vi "NIMS_dfd_Convert Band Specs (Remez Ripple).vi"(9 "Ripple":dbl[](array[numeric]), 10 "A":dbl[](array[numeric]), 11 "F":dbl[](array[numeric])) -> (0 "error out":errorcluster, 2 "band specs":T1[](array[typedef])=[{"band specification"=[{"freq"=0.0, "amplitude"=1.0, "weight"=1.0}, {"freq"=0.2, "amplitude"=1.0, "weight"=1.0}], "ripple constraint"=0.0}, {"band specification"=[{"freq"=0.3, "amplitude"=0.0, "weight"=1.0}, {"freq"=0.5, "amplitude"=0.0, "weight"=1.0}], "ripple constraint"=0.0}])   [LabVIEW 2017, in "NI_DigFilter_MathScript.lvlib"]
uses:
  <vilib>/addons/Digital Filter Design/NI_DigFilter_MathScript.lvlib
  <vilib>/addons/Digital Filter Design/_Objects.llb/DFD Adv Band Spec.ctl
  <vilib>/addons/Digital Filter Design/_Misc.llb/dfd_Error Handlers (Multiple).vi
  <vilib>/addons/Digital Filter Design/NI_DigFilterLicensed.lvlib
panel:
  # "freq"
  # "amplitude"
  # "weight"
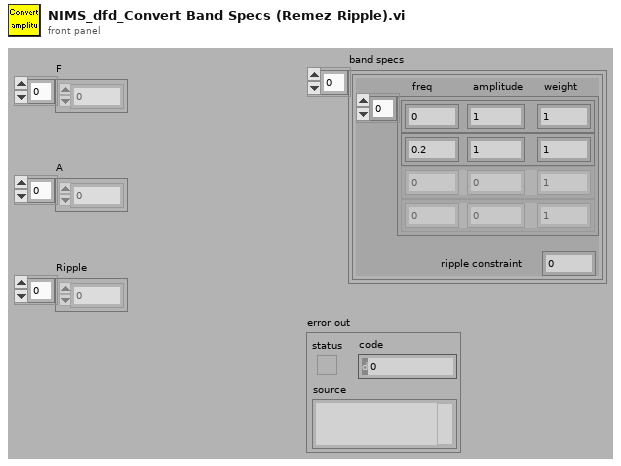
[diagram p1: front panel]
types:
  T1 = typedef "NI_DigFilterLicensed.lvlib/DFD Adv Band Spec.ctl" = cluster{"band specification":cluster{"freq":dbl, "amplitude":dbl, "weight":dbl}[], "ripple constraint":dbl}
  T2 = cluster{cluster{"Numeric":dbl, "Numeric":dbl, "x":dbl}[], "Numeric":dbl}
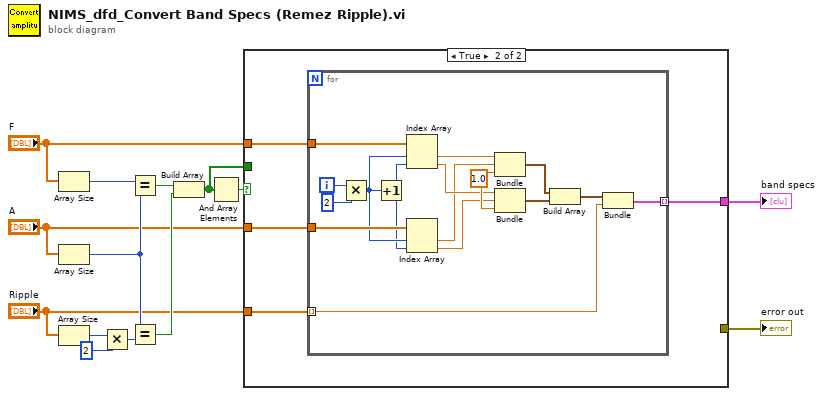
[diagram p0: block diagram]
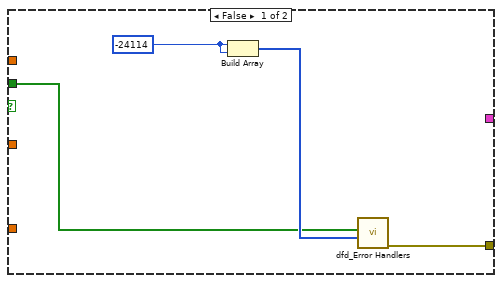
[diagram p2: hidden frame]
diagram:
  n1 = Array Size(array="F") -> (size(s)=w14:i32)
  n2 = Array Size(array="A") -> (size(s)=w12:i32)
  n3 = Array Size(array="Ripple") -> (size(s)=w4:i32)
  n4 = Multiply(x=w4, y=2) -> (x*y=w13:i32)
  n5 = Equal?(x=w14, y=w12) -> (x = y?=w11:bool)
  n6 = Equal?(x=w12, y=w13) -> (x = y?=w10:bool)
  n7 = Build Array(w11, w10) -> (w1:bool[])
  n8 = And Array Elements(Boolean array=w1) -> (logical AND=w2:bool)
  n9 = case shown="True" w2 {
    tunnel: "F" -> [_ w20]
    tunnel: "A" -> [_ w19]
    tunnel: "Ripple" -> [_ w22]
    tunnel: [_ w21] -> w6
    tunnel: [w16 _] -> w5
    tunnel: w1 -> [w15 _]
    frame False {
      w17 = -24114 ("element")
      n10 = Build Array(w17, w17) -> (w18:i32[])
      n11 = call-poly <vilib>:"dfd_Error Handlers.vi"("error sources"=w18, "condition failed?"=w15) -> ("error out"=w16:errorcluster)  [unwired: 1 in, 8 out]
    }
    frame True {
      n12 = for {
        tunnel: w22 -> [w33] mode=indexing
        tunnel: w20 -> [w32]
        tunnel: w19 -> [w31]
        tunnel: [w34] -> w21 mode=indexing
        i -> [w26]
        w38 = 1.0 ("x")
        n13 = Multiply(x=w26, y=2) -> (x*y=w24:i32)
        n14 = Increment(x=w24) -> (x+1=w23:i32)
        n15 = Index Array(array=w32, index #1=w24, index #2=w23) -> (element #1=w30:dbl, element #2=w29:dbl)
        n16 = Index Array(array=w31, index #1=w24, index #2=w23) -> (element #1=w28:dbl, element #2=w27:dbl)
        n17 = Bundle("Numeric"=w30, "Numeric"=w28, "x"=w38) -> (w37:cluster{"Numeric":dbl, "Numeric":dbl, "x":dbl})  [unwired: 1 out]
        n18 = Bundle("Numeric"=w29, "Numeric"=w27, "x"=w38) -> (w36:cluster{"Numeric":dbl, "Numeric":dbl, "x":dbl})  [unwired: 1 out]
        n19 = Build Array(w37, w36) -> (w35:cluster{"Numeric":dbl, "Numeric":dbl, "x":dbl}[])
        n20 = Bundle(w35, "Numeric"=w33) -> (w34:T2)  [unwired: 1 out]
      }
    }
  }
  "band specs" <- w6
  "error out" <- w5
